vi "LWXPS_GatheringCurrentNumberGet.vi"(0 "XPS Reference IN":refnum<k24>, 5 "LabVIEW error IN":errorcluster) -> (14 "XPS Reference OUT":refnum<k24>, 15 "Returned error code":i32, 16 "Current Number":i32, 17 "Maximum Samples Number":i32, 18 "XPS Error String":string, 19 "LabVIEW error OUT":errorcluster)   [LabVIEW 2014]
uses:
  D:/XPSQ8_LabView_Library/Development/Source/Dll/Newport.XPS.CommandInterface.dll
  Dll/Newport.XPS.CommandInterface.dll
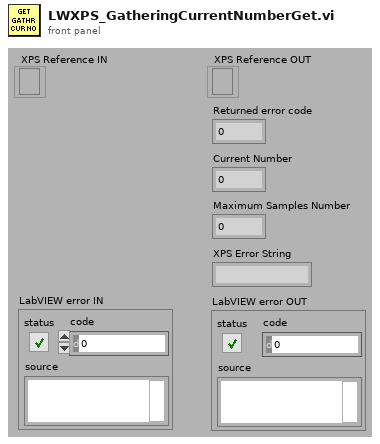
[diagram p1: front panel]
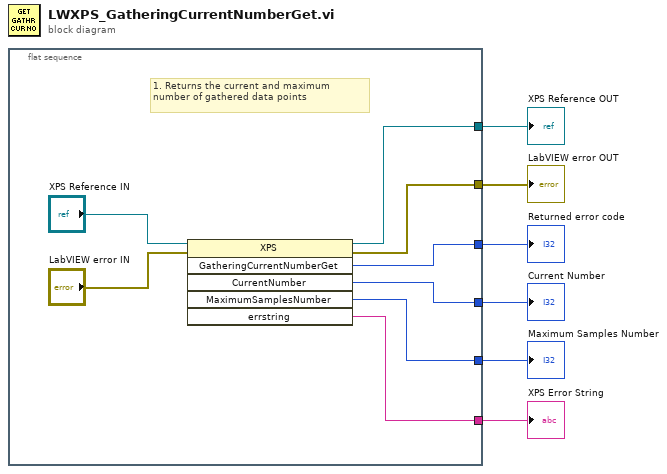
[diagram p0: block diagram]
diagram:
  n1 = flat-sequence {
    tunnel: [w13] -> w6
    tunnel: [w12] -> w5
    tunnel: [w11] -> w4
    tunnel: [w9] -> w2
    tunnel: [w8] -> w3
    tunnel: [w7] -> w1
    frame #0 {
      # "1. Returns the current and maximum number of gathered data points"
      n2 = invoke class="XPS" method="GatheringCurrentNumberGet"(reference="XPS Reference IN", error in="LabVIEW error IN") -> (reference out=w13:refnum<k24>, error out=w12:errorcluster, "GatheringCurrentNumberGet"=w11:i32, "CurrentNumber"=w9:i32, "MaximumSamplesNumber"=w7:i32, "errstring"=w8:string)  [unwired: 4 in]
    }
  }
  "XPS Reference OUT" <- w6
  "LabVIEW error OUT" <- w5
  "Returned error code" <- w4
  "XPS Error String" <- w3
  "Current Number" <- w2
  "Maximum Samples Number" <- w1
